vi "Remove Image From ImageList.vi"(8 "error in (no error)":errorcluster caption="错误输入（无错误）", 10 "index":i32, 11 "ImageListClass 输入":refnum<class "ImageListClass.lvclass"> caption="DNL_LabVIEW Object in") -> (0 "error out":errorcluster caption="错误输出", 3 "ImageListClass 输出":refnum<class "ImageListClass.lvclass"> caption="DNL_LabVIEW Object out")   [LabVIEW 2013, in "ImageListClass.lvclass"]
uses:
  ImageListClass.lvclass
  ImageListClass.lvclass/ImageListClass.ctl
  System.Windows.Forms
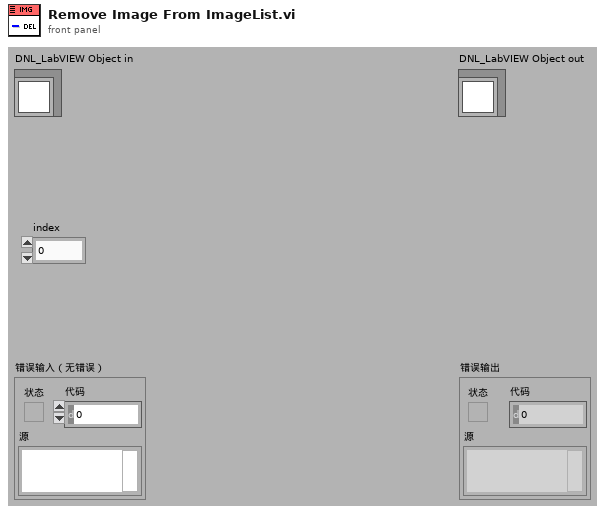
[diagram p1: front panel]
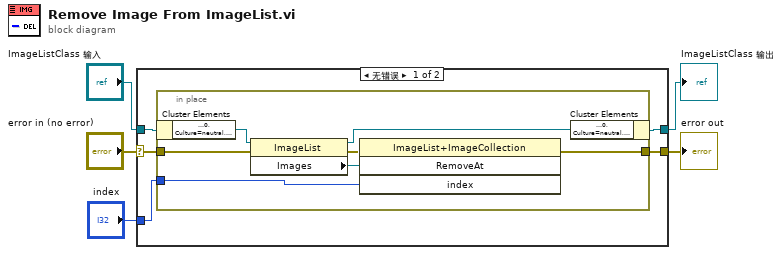
[diagram p0: block diagram]
diagram:
  n1 = case shown="无错误" "error in (no error)" {
    selector: "error in (no error)" -> [w7 w19]
    tunnel: [w6 w19] -> w4
    tunnel: [w8 w18] -> w2
    tunnel: "ImageListClass 输入" -> [w10 w18]
    tunnel: "index" -> [w9 _]
    frame No Error {
      n2 = in-place {
        in-place-border: w9 -> [w15]
        in-place-border: w7 -> [w13]
        in-place-border: [w11] -> w6
        n3 = in-place-cluster #1(w10) -> ("ImageList"=w17:refnum<k24>)
        n4 = property class="ImageList"(reference=w17, error in=w13) -> (reference out=w14:refnum<k24>, error out=w12:errorcluster, "Images"=w16:refnum<k24>)
        n5 = invoke class="ImageList+ImageCollection" method="RemoveAt"(reference=w16, error in=w12, "index"=w15) -> (error out=w11:errorcluster)  [unwired: 1 in, 3 out]
        n6 = in-place-cluster #1("ImageList"=w14) -> (w8:refnum<class "ImageListClass.lvclass">)
      }
    }
    frame Error {
    }
  }
  "error out" <- w4
  "ImageListClass 输出" <- w2
